vi "Stop.vi"(8 "error in":errorcluster, 11 "IModulate Voltage in":refnum<class "IModulate Voltage.lvclass">) -> (0 "error out":errorcluster, 3 "IModulate Voltage out":refnum<class "IModulate Voltage.lvclass">)   [LabVIEW 2023, in "HAL Interfaces.lvlib" / "IModulate Voltage.lvclass"]
uses:
  IModulate Voltage.lvclass
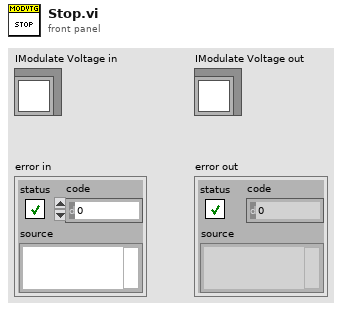
[diagram p1: front panel]
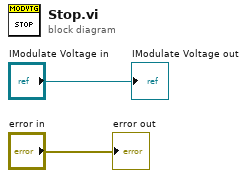
[diagram p0: block diagram]
diagram:
  "error out" <- "error in"
  "IModulate Voltage out" <- "IModulate Voltage in"
